vi "Framework Host Sobot.vi"() -> ()   [LabVIEW 2017]
uses:
  TypeDefinitions/TCP Cluster.ctl
  TypeDefinitions/TCP Commands.ctl
  TypeDefinitions/Sobot Driving Data.ctl
  <vilib>/Utility/inputDevices.llb/closeJoystick.vi
  <vilib>/Instr/_visa.llb/VISA Configure Serial Port (Instr).vi
panel:
  out "value":T1
  out "Driving Data":u8[](array[numeric])
  in  "stop 2":bool
  in  "device index":i32
  in  "Manuelles Fahren (Joystick)":bool
  in  "VISA resource name":refnum<visa-resource-name>
  out "Send":T2={"Datatype"=enum."Message", "String"="Send to sobot"}
  out "Receive":T2={"Datatype"=enum."Message", "String"="Send to sobot"}
  in  "Button 2":bool
  in  "stop":bool
  in  "Button 1":bool
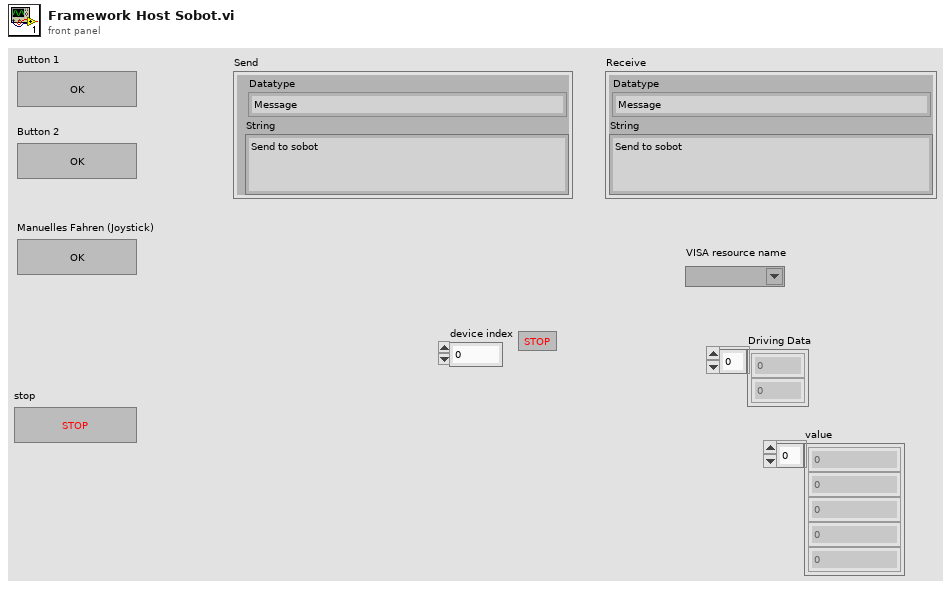
[diagram p1: front panel]
types:
  T1 = typedef "Sobot Driving Data.ctl" = u8[]
  T2 = typedef "TCP Cluster.ctl" = cluster{"Datatype":T3, "String":string}
  T3 = typedef "TCP Commands.ctl" = enum16{"Message", "sobotManualDrive", "Stop", "Command"}
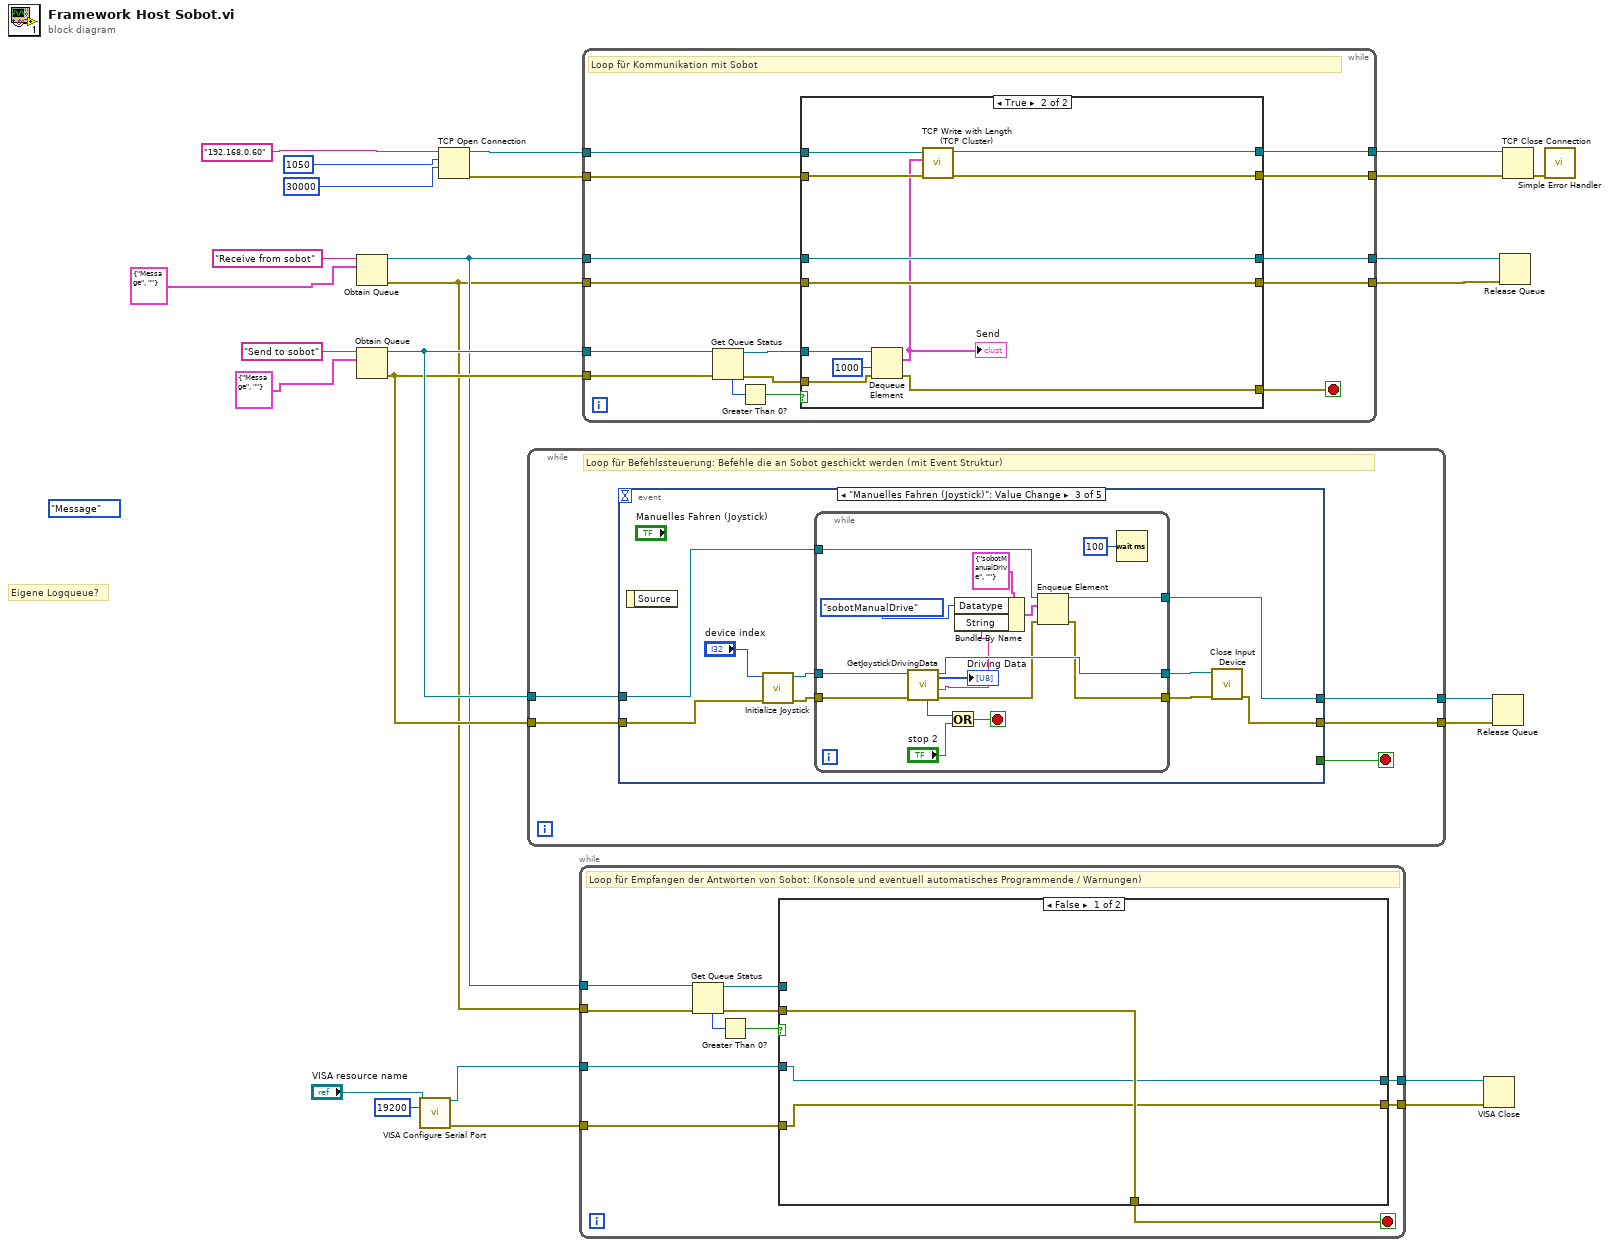
[diagram p0: block diagram]
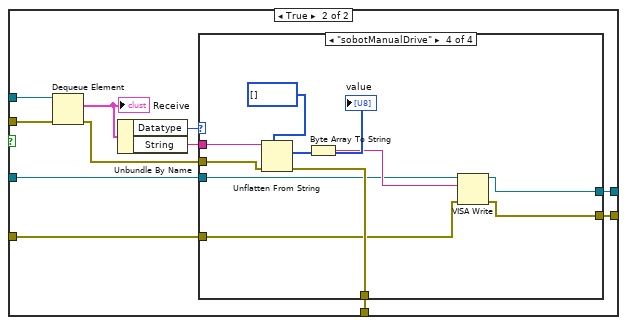
[diagram p2: hidden frame]
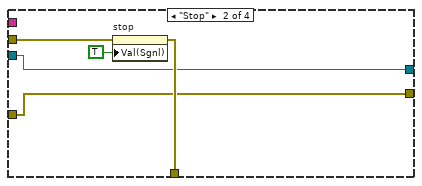
[diagram p4: hidden frame]
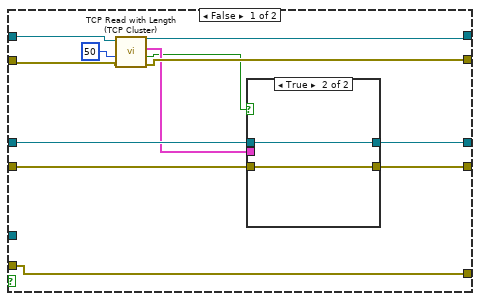
[diagram p6: hidden frame]
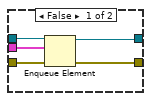
[diagram p7: hidden frame]
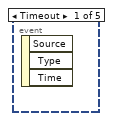
[diagram p8: hidden frame]
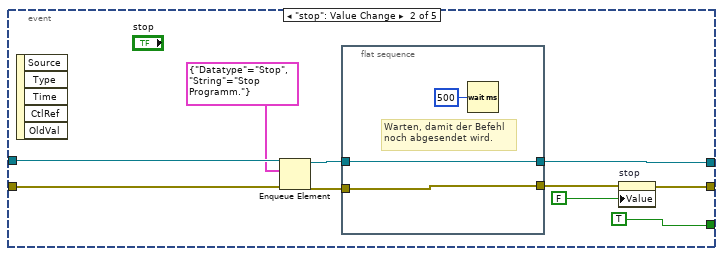
[diagram p9: hidden frame]
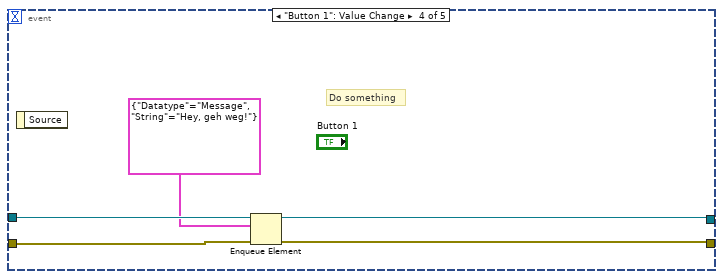
[diagram p10: hidden frame]
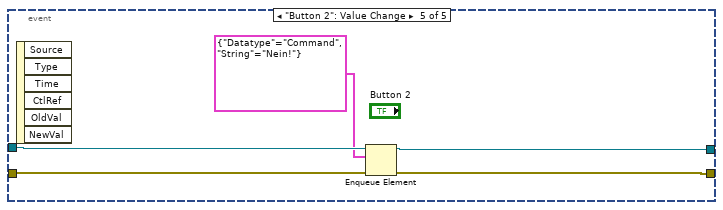
[diagram p11: hidden frame]
diagram:
  (unwired) TCP_Commands."Message"
  # "Eigene Logqueue?"
  n1 = Obtain Queue(name (unnamed)="Receive from sobot", element data type=T2 {"Datatype"=enum."Message", "String"=""}) -> (queue out=w17:refnum<queue>, error out=w16:errorcluster)  [unwired: 3 in, 1 out]
  n2 = Obtain Queue(name (unnamed)="Send to sobot", element data type=T2 {"Datatype"=enum."Message", "String"=""}) -> (queue out=w25:refnum<queue>, error out=w22:errorcluster)  [unwired: 3 in, 1 out]
  n3 = call-poly "VISA Configure Serial Port"("VISA resource name"="VISA resource name", "baud rate (9600)"=u32 19200) -> ("VISA resource name out"=w7:refnum<visa-resource-name>, "error out"=w6:errorcluster)  [unwired: 12 in]
  n4 = TCP Open Connection(address="192.168.0.60", remote port or service name=u16 1050, timeout ms (60000)=30000) -> (connection ID=w5:refnum<k5>, error out=w4:errorcluster)  [unwired: 2 in]
  n5 = while {
    tunnel: w25 -> [w30]
    tunnel: [w29] -> w24
    tunnel: [w28] -> w23
    tunnel: w22 -> [w27]
    stop <- w31 stop-if-true
    # "Loop für Befehlssteuerung: Befehle die an Sobot geschickt werden (mit Event Struktur)"
    n6 = event shown="[2] \"Manuelles Fahren (Joystick)\": Value Change" {
      selector: _ -> [_ _ _ _ _]
      dyn-events: _ -> [_ _ _ _ _]
      timeout: _ -> [_ _ _ _ _]
      tunnel: [_ TRUE _ _ _] -> w31
      tunnel: w30 -> [_ w40 w46 w74 w79]
      tunnel: [_ w36 w45 w71 w78] -> w29
      tunnel: [_ w33 w47 w72 w77] -> w28
      tunnel: w27 -> [_ w39 w48 w73 w76]
      event Timeout {
        n7 = event-data() -> ()  [unwired: 1 in, 3 out]
      }
      event "stop": Value Change {
        n8 = event-data() -> ()  [unwired: 1 in, 5 out]
        n9 = Enqueue Element(queue=w40, element=T2 {"Datatype"=enum."Stop", "String"="Stop Programm."}, error in (no error)=w39) -> (queue out=w37:refnum<queue>, error out=w35:errorcluster)  [unwired: 1 in, 1 out]
        n10 = flat-sequence {
          tunnel: w37 -> [w44]
          tunnel: [w44] -> w36
          tunnel: [w42] -> w34
          tunnel: w35 -> [w42]
          frame #0 {
            # "Warten, damit der Befehl\nnoch abgesendet wird."
            n11 = Wait (ms)(milliseconds to wait=u32 500) -> ()  [unwired: 1 out]
          }
        }
        n12 = property on="stop" class="Bool (strict)"(error in=w34, "Value"=FALSE ("stop")) -> (error out=w33:errorcluster)  [unwired: 1 in, 1 out]
      }
      event "Manuelles Fahren (Joystick)": Value Change {
        n13 = event-data() -> ()  [unwired: 1 in, 1 out]
        n14 = call <vilib>:"Initialize Joystick.vi"("error in (no error)"=w48, "device index"="device index") -> ("error out"=w52:errorcluster, "device ID"=w53:refnum<k1>)  [unwired: 8 in]
        n15 = while {
          tunnel: w53 -> [w69]
          tunnel: w52 -> [w68]
          tunnel: [w67] -> w50
          tunnel: [w55] -> w49
          tunnel: w46 -> [w58]
          tunnel: [w57] -> w45
          stop <- w64 stop-if-true
          n16 = call "GetJoystickDrivingData.vi"("error in (no error)"=w68, "Refnum in"=w69) -> ("error out"=w56:errorcluster, "data string"=w61:string, "Refnum out"=w67:refnum<k1>, "Boolean"=w65:bool, "Array"=→"Driving Data":u8[])  [unwired: 4 in, 1 out]
          n17 = Or(x=w65, y="stop 2") -> (x .or. y?=w64:bool)
          n18 = Bundle By Name(cluster=T2 {"Datatype"=enum."sobotManualDrive", "String"=""}, "Datatype"=TCP_Commands."sobotManualDrive", "String"=w61) -> (w59:T2)
          n19 = Enqueue Element(queue=w58, element=w59, error in (no error)=w56) -> (queue out=w57:refnum<queue>, error out=w55:errorcluster)  [unwired: 1 in, 1 out]
          n20 = Wait (ms)(milliseconds to wait=u32 100) -> ()  [unwired: 1 out]
        }
        n21 = call-poly <vilib>:"Close Input Device.vi"("error in (no error)"=w49, "device ID"=w50) -> ("error out"=w47:errorcluster)  [unwired: 8 in]
      }
      event "Button 1": Value Change {
        # "Do something"
        n22 = event-data() -> ()  [unwired: 1 in, 1 out]
        n23 = Enqueue Element(queue=w74, element=T2 {"Datatype"=enum."Message", "String"="Hey, geh weg!"}, error in (no error)=w73) -> (queue out=w71:refnum<queue>, error out=w72:errorcluster)  [unwired: 1 in, 1 out]
      }
      event "Button 2": Value Change {
        n24 = event-data() -> ()  [unwired: 1 in, 6 out]
        n25 = Enqueue Element(queue=w79, element=T2 {"Datatype"=enum."Command", "String"="Nein!"}, error in (no error)=w76) -> (queue out=w78:refnum<queue>, error out=w77:errorcluster)  [unwired: 1 in, 1 out]
      }
    }
  }
  n26 = while {
    tunnel: w17 -> [w89]
    tunnel: w16 -> [w88]
    tunnel: [w83] -> w11
    tunnel: [w82] -> w10
    tunnel: w7 -> [w81]
    tunnel: w6 -> [w80]
    stop <- w84 stop-if-true
    # "Loop für Empfangen der Antworten von Sobot: (Konsole und eventuell automatisches Programmende / Warnungen)"
    n27 = Get Queue Status(queue=w89, error in (no error)=w88) -> (queue out=w86:refnum<queue>, error out=w85:errorcluster, # elements in queue=w90:i32)  [unwired: 1 in, 5 out]
    n28 = Greater Than 0?(x=w90) -> (x > 0?=w87:bool)
    n29 = case shown="False" w87 {
      tunnel: w86 -> [_ w104]
      tunnel: w85 -> [w93 w103]
      tunnel: [w93 w99] -> w84
      tunnel: [w91 w97] -> w83
      tunnel: [w92 w96] -> w82
      tunnel: w81 -> [w92 w95]
      tunnel: w80 -> [w91 w94]
      frame False {
      }
      frame True {
        n30 = Dequeue Element(queue=w104, error in (no error)=w103) -> (element=w102:T2, error out=w100:errorcluster)  [unwired: 1 in, 2 out]
        "Receive" <- w102
        n31 = Unbundle By Name(w102) -> ("Datatype"=w101:T3, "String"=w98:string)
        n32 = case shown="\"sobotManualDrive\"" w101 {
          tunnel: w100 -> [w107 w111 w115 w123]
          tunnel: [w107 w110 w115 w122] -> w99
          tunnel: w98 -> [_ _ _ w125]
          tunnel: [w105 w108 w113 w119] -> w97
          tunnel: [w106 w109 w114 w118] -> w96
          tunnel: w95 -> [w106 w109 w114 w117]
          tunnel: w94 -> [w105 w108 w113 w116]
          frame "Message", Default {
          }
          frame "Stop" {
            n33 = property on="stop" class="Bool (strict)"(error in=w111, "Val(Sgnl)"=TRUE ("Value (Signaling)")) -> (error out=w110:errorcluster)  [unwired: 1 in, 1 out]
          }
          frame "Command" {
          }
          frame "sobotManualDrive" {
            n34 = Unflatten From String(type=T1 [] ("Sobot Driving Data"), binary string=w125, error in (no error)=w123) -> (value=w121:T1, error out=w122:errorcluster)  [unwired: 2 in, 1 out]
            "value" <- w121
            n35 = Byte Array To String(unsigned byte array=w121) -> (string=w120:string)
            n36 = VISA Write(VISA resource name=w117, write buffer=w120, error in (no error)=w116) -> (VISA resource name out=w118:refnum<visa-resource-name>, error out=w119:errorcluster)  [unwired: 1 out]
          }
        }
      }
    }
  }
  n37 = while {
    tunnel: w25 -> [w139]
    tunnel: w22 -> [w137]
    tunnel: w5 -> [w133]
    tunnel: w4 -> [w132]
    tunnel: [w131] -> w20
    tunnel: [w130] -> w19
    tunnel: w17 -> [w129]
    tunnel: w16 -> [w128]
    tunnel: [w127] -> w14
    tunnel: [w126] -> w15
    stop <- w140 stop-if-true
    # "Loop für Kommunikation mit Sobot"
    n38 = Get Queue Status(queue=w139, error in (no error)=w137) -> (queue out=w138:refnum<queue>, error out=w136:errorcluster, # elements in queue=w135:i32)  [unwired: 1 in, 5 out]
    n39 = Greater Than 0?(x=w135) -> (x > 0?=w134:bool)
    n40 = case shown="True" w134 {
      tunnel: [w152 w170] -> w140
      tunnel: w138 -> [_ w168]
      tunnel: w136 -> [w152 w167]
      tunnel: w133 -> [w147 w164]
      tunnel: w132 -> [w146 w163]
      tunnel: [w144 w162] -> w130
      tunnel: [w143 w161] -> w131
      tunnel: w129 -> [w151 w166]
      tunnel: w128 -> [w150 w165]
      tunnel: [w149 w166] -> w126
      tunnel: [w148 w165] -> w127
      frame False {
        n41 = call "TCP Read with Length (TCP Cluster).vi"("error in (no error)"=w146, "Timeout"=50, "connection ID"=w147) -> ("error out"=w144:errorcluster, "Timeout?"=w141:bool, "TCP Cluster"=w142:T2, "connection ID out"=w143:refnum<k5>)  [unwired: 5 in]
        n42 = case shown="True" w141 {
          tunnel: w151 -> [w157 w159]
          tunnel: w150 -> [w156 w158]
          tunnel: w142 -> [w155 _]
          tunnel: [w154 w159] -> w149
          tunnel: [w153 w158] -> w148
          frame False {
            n43 = Enqueue Element(queue=w157, element=w155, error in (no error)=w156) -> (queue out=w154:refnum<queue>, error out=w153:errorcluster)  [unwired: 1 in, 1 out]
          }
          frame True {
          }
        }
      }
      frame True {
        n44 = Dequeue Element(queue=w168, timeout in ms (-1)=1000, error in (no error)=w167) -> (element=w160:T2, error out=w170:errorcluster)  [unwired: 2 out]
        "Send" <- w160
        n45 = call "TCP Write with Length (TCP Cluster).vi"("error in (no error)"=w163, 10:w160, "connection ID"=w164) -> ("error out"=w162:errorcluster, "connection ID out"=w161:refnum<k5>)  [unwired: 7 in]
      }
    }
  }
  n46 = VISA Close(VISA resource name=w10, error in (no error)=w11) -> ()  [unwired: 1 out]
  n47 = Release Queue(queue=w24, error in (no error)=w23) -> ()  [unwired: 1 in, 3 out]
  n48 = Release Queue(queue=w15, error in (no error)=w14) -> ()  [unwired: 1 in, 3 out]
  n49 = TCP Close Connection(connection ID=w20, error in (no error)=w19) -> (error out=w21:errorcluster)  [unwired: 1 in, 1 out]
  n50 = call <vilib>:"Simple Error Handler.vi"("error in (no error)"=w21) -> ()  [unwired: 4 in, 5 out]
